vi "firewallLogs.vi"() -> ()   [LabVIEW 2014]
uses:
  <vilib>/regexp/Match Regular Expression.xnode
panel:
  in  "file path (use dialog)":path
  out "?":string[][](array[string])
  in  "input string":string="Apr 26 21:31:34 filterlog: 129,16777216,,1425041642,hn0,match,pass,in,4,0x0,,128,16110,0,none,17,udp,36,10.2.10.175,255.255.255.255,60221,3956,16\nApr 26 21:31:34 filterlog: 129,16777216,,1425041642,hn0,match,pass,in,4,0x0,,128,4117,0,none,17,udp,78,10.2.10.1,208.93.4.206,137,137,58\nApr 26 21:31:32 filterlog: 130,16777216,,1425041643,hn0,match,pass,in,4,0x0,,128,18168,0,DF,17,udp,351,10.2.10.10,10.2.23.123,53,59118,331\nApr 26 21:31:32 filterlog: 129,16777216,,1425041642,hn0,match,pass,in,4,0x0,,128,10627,0,none,17,udp,82,10.2.10.10,140.112.2.2,59087,53,62\nApr 26 21:31:32 filterlog: 129,16777216,,1425041642,hn0,match,pass,in,4,0x0,,128,10626,0,none,17,udp,98,10.2.10.10,140.112.2.2,60847,53,78\nApr 26 21:38:10 filterlog: 105,16777216,,1425041627,hn1,match,block,in,4,0x2,0,109,9812,0,DF,6,tcp,48,207.46.13.171,10.2.10.15,25309,80,0,SEC,27892632,,8192,,mss;nop;nop;sackOK\nApr 26 21:38:08 filterlog: 129,16777216,,1425041642,hn0,match,pass,in,4,0x0,,128,23124,0,DF,6,tcp,52,10.2.10.172,207.46.153.155,60590,443,0,S,2141064781,,8192,,mss;nop;wscale;nop;nop;sackOK\nApr 26 21:38:08 filterlog: 130,16777216,,1425041643,hn0,match,block,in,4,0x2,0,128,8596,0,DF,6,tcp,48,10.2.10.2,10.2.102.10,41875,88,0,SEC,3256166066,,8192,,mss;nop;nop;sackOK\nApr 26 21:38:07 filterlog: 130,16777216,,1425041643,hn0,match,pass,in,4,0x2,0,128,8592,0,DF,6,tcp,48,10.2.10.2,10.2.102.10,41874,88,0,SEC,2184502132,,8192,,mss;nop;nop;sackOK"
  # "Date-time            Interface-name         Pass-or-block       Internet Protocol       Packet Length      Protocol Source-ip         Target-ip               Source-port              Target-port"
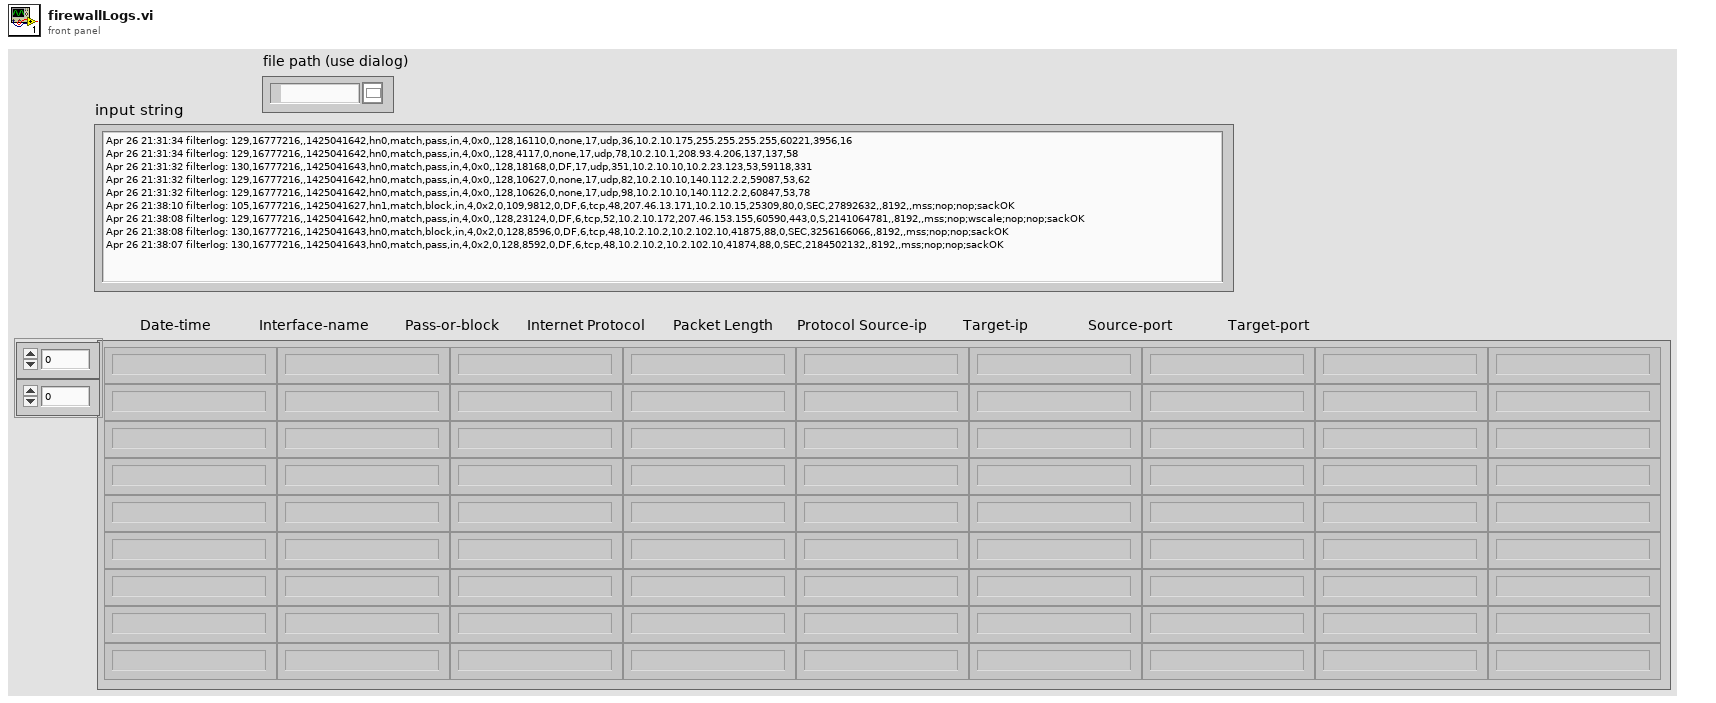
[diagram p1: front panel]
types:
  T1 = enum16{"open", "replace", "create", "open or create", "replace or create", "replace or create with confirmation"}
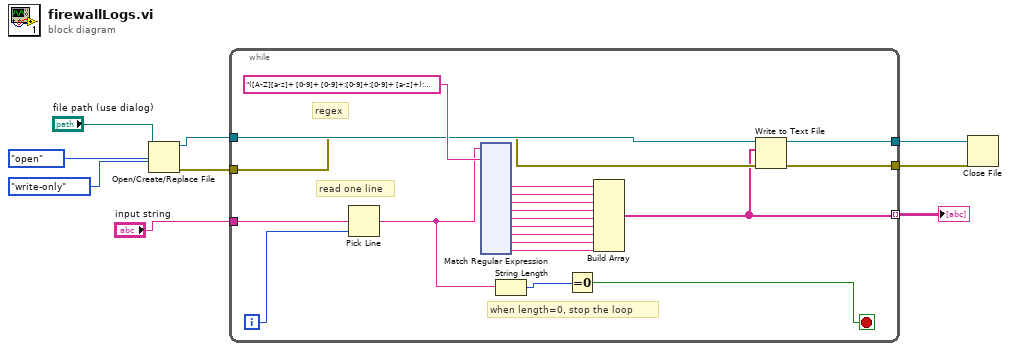
[diagram p0: block diagram]
diagram:
  n1 = Open/Create/Replace File(file path (use dialog)="file path (use dialog)", operation (0:open)=T1."open", access (0:read/write)=enum16{"read/write", "read-only", "write-only"}."write-only") -> (refnum out=w7:refnum<file>, error out=w6:errorcluster)  [unwired: 3 in, 1 out]
  n2 = while {
    tunnel: [w10] -> w9 mode=indexing
    tunnel: "input string" -> [w19]
    tunnel: w7 -> [w14]
    tunnel: w6 -> [w13]
    tunnel: [w12] -> w5
    tunnel: [w11] -> w4
    i -> [w18]
    stop <- w15 stop-if-true
    # "regex"
    # "when length=0, stop the loop"
    # "read one line"
    n3 = Pick Line(multi-line string=w19, line index=w18) -> (output string=w17:string)  [unwired: 1 in]
    n4 = xnode "Match Regular Expression"("input string"=w17, "regular expression"="([A-Z][a-z]+ [0-9]+ [0-9]+:[0-9]+:[0-9]+ [a-z]+): [0-9]+,[0-9]+,,[0-9]+,([a-z][a-z][0-9]),[a-z]+,([a-z]+),[a-z]+,[0-9],[0-9]x[0-9],[,0-9]+[0-9]+,[0-9]+,[0-9]+,[a-zA-Z]+,[0-9]+,([tu][cd]p),([0-9]+),([0-9]+.[0-9]+.[0-9]+.[0-9]+),([0-9]+.[0-9]+.[0-9]+.[0-9]+),([0-9]+),([0-9]+)") -> ("submatch 1"=w29:string, "submatch 2"=w28:string, "submatch 3"=w27:string, "submatch 4"=w26:string, "submatch 5"=w25:string, "submatch 6"=w24:string, "submatch 7"=w23:string, "submatch 8"=w22:string, "submatch 9"=w21:string)  [unwired: 4 in, 5 out]
    n5 = String Length(string=w17) -> (length=w16:i32)
    n6 = Equal To 0?(x=w16) -> (x = 0?=w15:bool)
    n7 = Build Array(w29, w28, w27, w26, w25, w24, w23, w22, w21) -> (w10:string[])
    n8 = Write to Text File(file (use dialog)=w14, text=w10, error in=w13) -> (refnum out=w11:refnum<file>, error out=w12:errorcluster)  [unwired: 1 in, 1 out]
  }
  "?" <- w9
  n9 = Close File(refnum=w4, error in=w5) -> ()  [unwired: 2 out]
